vi "ATM Controller Main.vi"(8 "error in (no error)":errorcluster) -> (0 "error out":errorcluster)   [LabVIEW 2020, in "ATM_Controller.lvlib"]
doc: "This is the Main VI for the ATM Controller Module."
uses:
  ATM_Controller.lvlib
  Private Controls/FG Actions.ctl
  Private Controls/Module Data.ctl
  Private Controls/Message Cluster.ctl
  Private Controls/Message enum.ctl
  User Console/User Console.lvlib
  Display Console/Display Console.lvlib
  Sensor Interface/Sensor Interface.lvlib
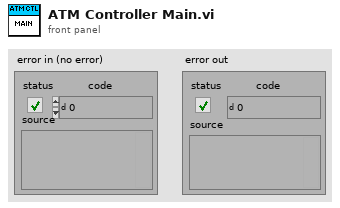
[diagram p1: front panel]
types:
  T1 = typedef "ATM_Controller.lvlib/Module Data.ctl" = cluster{"Data":variant}
  T2 = typedef "ATM_Controller.lvlib/FG Actions.ctl" = enum16{"Get", "Set", "Clear"}
  T3 = typedef "ATM_Controller.lvlib/Message Cluster.ctl" = cluster{"Message":T4, "Data":variant}
  T4 = typedef "ATM_Controller.lvlib/Message enum.ctl" = enum16{"Initialize", "State", "Error", "Exit", "Terminate", "Log In"}
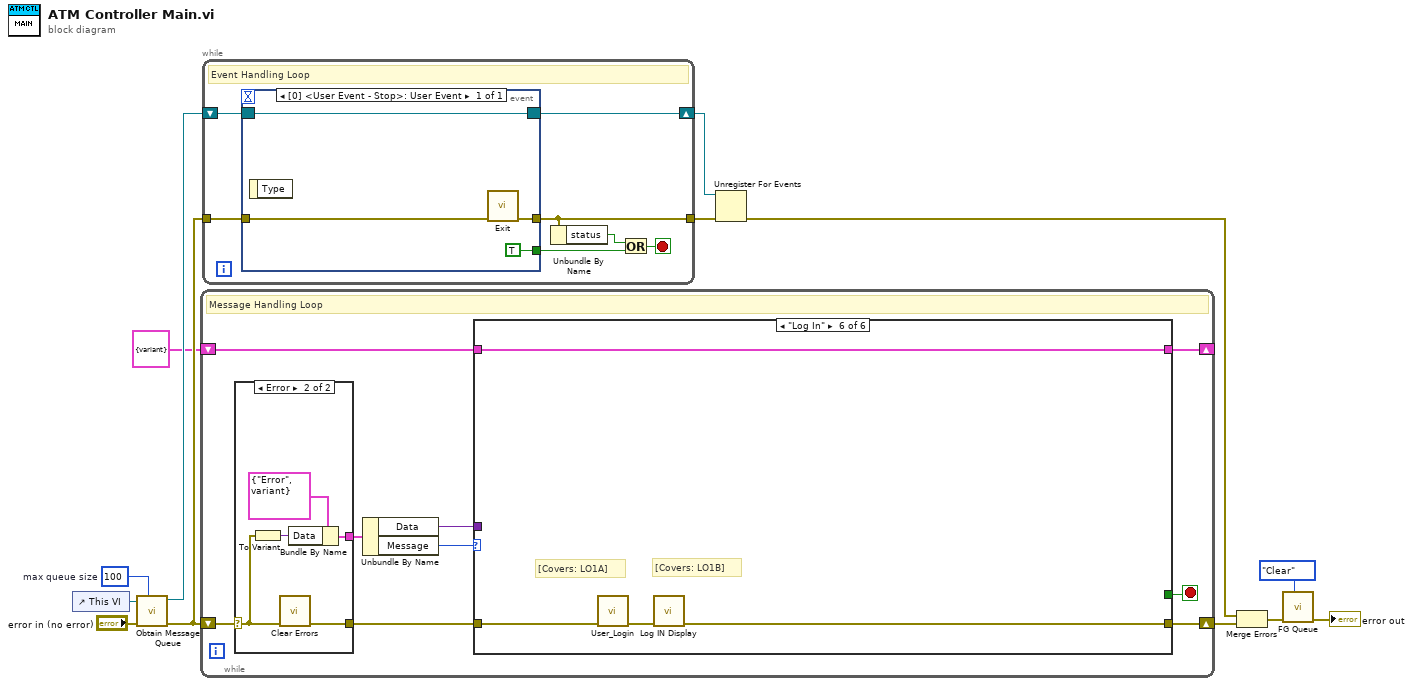
[diagram p0: block diagram]
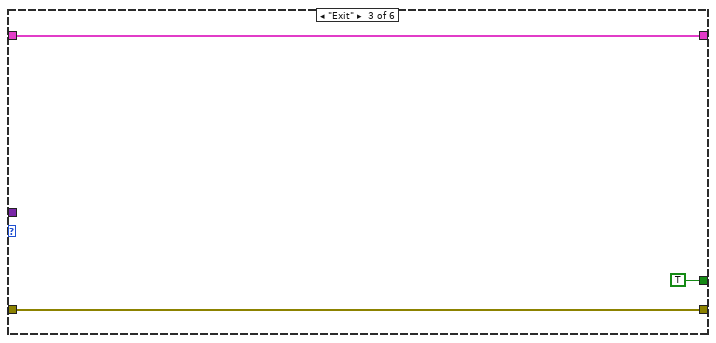
[diagram p4: hidden frame]
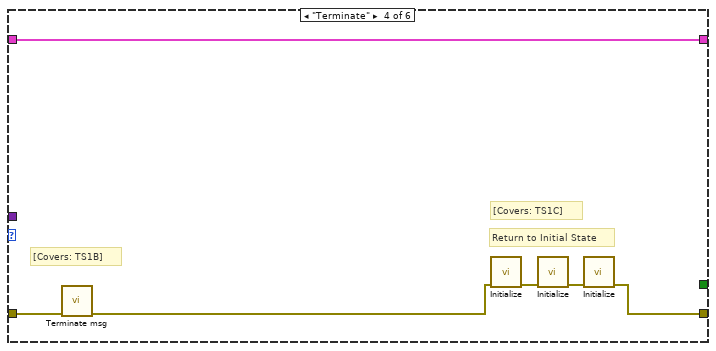
[diagram p5: hidden frame]
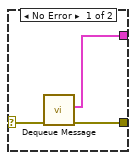
[diagram p7: hidden frame]
diagram:
  w7 = 100  # max queue size
  n1 = control-ref of="This VI"() -> (w8:refnum<vi>)
  n2 = call "Obtain Message Queue.vi"("max queue size (-1, unlimited)"=w7, "error in (no error)"="error in (no error)", "VI Reference"=w8) -> ("error out"=w3:errorcluster, "Event Registration Refnum"=w10:refnum<event-registration>)  [unwired: 7 in]
  n3 = while {
    shift-right: [w17] -> w13
    shift-left: w3 -> [w22]
    shift-right: [w14] -> _
    shift-left: T1 {"Data"=variant} ("Message Cluster") -> [w15]
    stop <- w16 stop-if-true
    # "Message Handling Loop"
    n4 = case shown="Error" w22 {
      selector: w22 -> [w42 w48]
      tunnel: [w43 w49] -> w18
      tunnel: [w44 w45] -> w21
      frame No Error {
        n5 = call "Dequeue Message.vi"("error in (no error)"=w42) -> ("error out"=w43:errorcluster, "Element"=w44:T3)  [unwired: 9 in]
      }
      frame Error {
        n6 = To Variant(anything=w48) -> (Variant=w46:variant)
        n7 = call <vilib>:"Clear Errors.vi"("error in (no error)"=w48) -> ("error out"=w49:errorcluster)  [unwired: 5 in, 1 out]
        n8 = Bundle By Name(cluster=T3 {"Message"=enum."Error", "Data"=variant} ("Message Cluster"), "Data"=w46) -> (w45:T3)
      }
    }
    n9 = Unbundle By Name(w21) -> ("Data"=w19:variant, "Message"=w20:T4)
    n10 = case shown="\"Log In\"" w20 {
      tunnel: w19 -> [_ _ _ _ _ _]
      tunnel: w18 -> [w24 w26 w29 w31 w37 w40]
      tunnel: [w24 w26 w29 w32 w37 w38] -> w17
      tunnel: [_ _ TRUE _ _ _] -> w16
      tunnel: w15 -> [w23 w25 w27 w35 w36 w41]
      tunnel: [w23 w25 w27 w35 w36 w41] -> w14
      frame "Initialize", Default {
      }
      frame "Error" {
      }
      frame "Exit" {
      }
      frame "Terminate" {
        # "[Covers: TS1B]"
        # "Return to Initial State"
        # "[Covers: TS1C]"
        n11 = call "Terminate msg.vi"("error in (no error)"=w31) -> ("error out"=w30:errorcluster)  [unwired: 10 in]
        n12 = call "Initialize.vi"("error in (no error)"=w30) -> ("error out"=w34:errorcluster)  [unwired: 10 in]
        n13 = call "Initialize.vi"("error in (no error)"=w34) -> ("error out"=w33:errorcluster)  [unwired: 10 in]
        n14 = call "Initialize.vi"("error in (no error)"=w33) -> ("error out"=w32:errorcluster)  [unwired: 10 in]
      }
      frame "State" {
      }
      frame "Log In" {
        # "[Covers: LO1B]"
        # "[Covers: LO1A]"
        n15 = call "User_Login.vi"("error in (no error)"=w40) -> ("error out"=w39:errorcluster)  [unwired: 10 in]
        n16 = call "Log IN Display.vi"("error in (no error)"=w39) -> ("error out"=w38:errorcluster)  [unwired: 10 in]
      }
    }
  }
  n17 = while {
    shift-right: [w55] -> w11
    shift-left: w10 -> [w56]
    tunnel: w3 -> [w53]
    tunnel: [w51] -> w2
    stop <- w52 stop-if-true
    # "Event Handling Loop"
    n18 = event shown="[0] <User Event - Stop>: User Event" {
      selector: w56 -> [w57]
      dyn-events: [w57] -> w55
      timeout: _ -> [_]
      tunnel: [TRUE ("Discard?")] -> w54
      tunnel: w53 -> [w59]
      tunnel: [w58] -> w51
      event User Event {
        n19 = event-data() -> ()  [unwired: 1 in, 1 out]
        n20 = call "Exit.vi"("error in (no error)"=w59) -> ("error out"=w58:errorcluster)  [unwired: 10 in]
      }
    }
    n21 = Unbundle By Name(w51) -> ("status"=w50:bool)
    n22 = Or(x=w50, y=w54) -> (x .or. y?=w52:bool)
  }
  n23 = Unregister For Events(event registration refnum=w11, error in=w2) -> (error out=w12:errorcluster)
  n24 = Merge Errors(w12, w13) -> (w5:errorcluster)
  n25 = call "FG Queue.vi"("FG Actions"=FG_Actions."Clear", "error in (no error)"=w5) -> ("error out"=→"error out":errorcluster)  [unwired: 8 in, 1 out]
